vi "PopulateControlsFromCSV-OLD.vi"() -> ()   [LabVIEW 2019]
uses:
  <vilib>/Utility/file.llb/Read Delimited Spreadsheet (string).vi
panel:
  out "Boolean":bool
  out "number":dbl
  out "element":string
  out "index of element":i32
  out "Label.Text":string="all rows"
  out "all rows":string[][](array[string])
  in  "Numeric4":dbl
  in  "Numeric3":dbl
  in  "Numeric2":dbl
  in  "Numeric1":dbl
  in  "Path":path=path "C:/Users/jbrus/Documents/GitHub/LabVIEW/3LabVIEWFeatures/PopulateControlsFromCSV/FileOutput.csv"
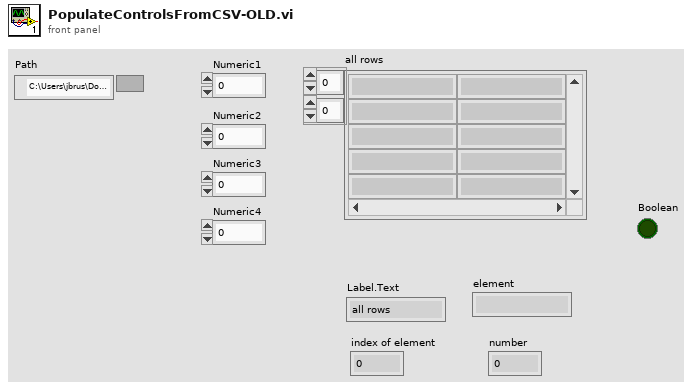
[diagram p1: front panel]
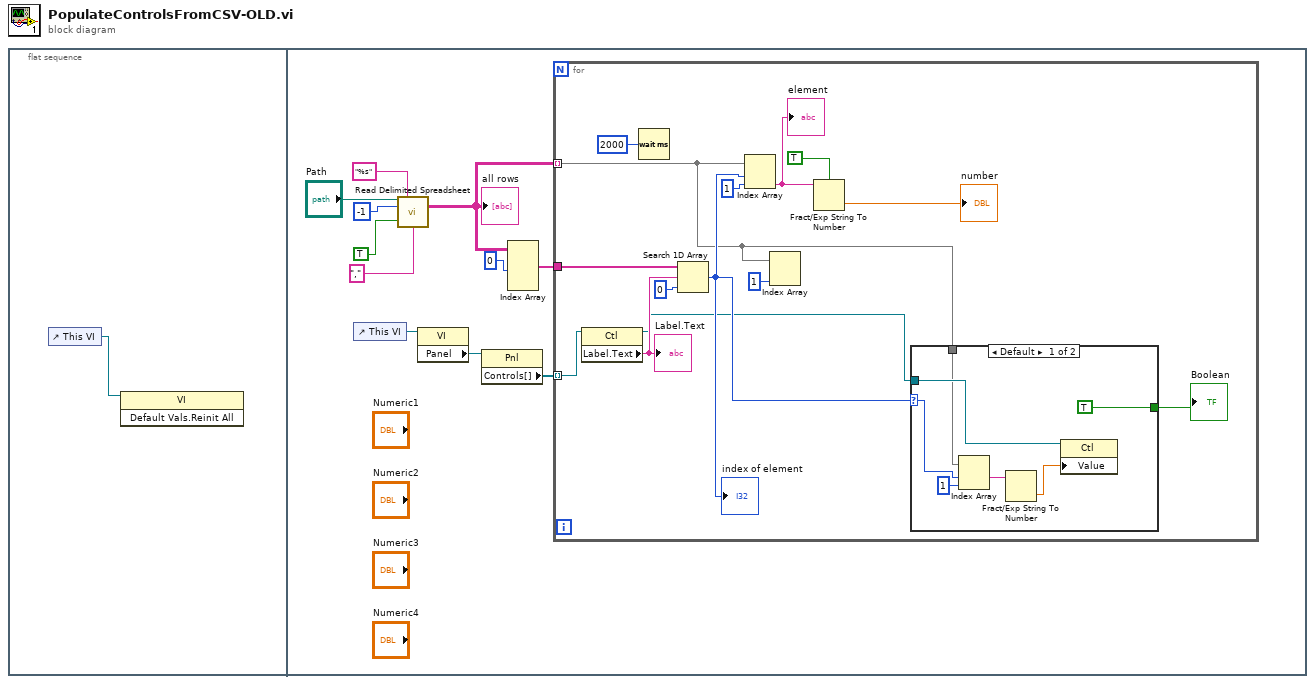
[diagram p0: block diagram]
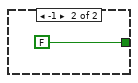
[diagram p2: hidden frame]
diagram:
  n1 = flat-sequence {
    frame #0 {
      n2 = control-ref of="This VI"() -> (w1:refnum<vi>)
      n3 = invoke class="VI" method="Default Vals.Reinit All"(reference=w1) -> ()  [unwired: 2 in, 3 out]
    }
    frame #1 {
      n4 = control-ref of="This VI"() -> (w7:refnum<vi>)
      n5 = call-poly <vilib>:"Read Delimited Spreadsheet.vi"("file path (dialog if empty)"="Path", "format (%s)"="%s", "number of rows (all:-1)"=-1, "transpose? (F)"=TRUE, "delimiter (\\t)"="," ("delimiter (\\t)")) -> ("all rows"=w12:string[][])  [unwired: 5 in, 5 out]
      "all rows" <- w12
      n6 = property class="VI"(reference=w7) -> ("Panel"=w8:refnum<vi>)  [unwired: 1 in, 2 out]
      n7 = property class="Pnl"(reference=w8) -> ("Controls[]"=w9:refnum<vi>[])  [unwired: 1 in, 2 out]
      n8 = Index Array(array=w12, index (col) #1=0 ("index")) -> (element #1=w11:string[])  [unwired: 3 in, 1 out]
      n9 = for {
        tunnel: w9 -> [w16] mode=indexing
        tunnel: w11 -> [w24]
        tunnel: w12 -> [w14] mode=indexing
        n10 = property class="Ctl"(reference=w16) -> (reference out=w13:refnum<vi>, "Label.Text"=w23:string)  [unwired: 1 in, 1 out]
        "Label.Text" <- w23
        n11 = Wait (ms)(milliseconds to wait=u32 2000) -> ()  [unwired: 1 out]
        n12 = Search 1D Array(1D array=w24, element=w23, start index (0)=0) -> (index of element=w18:i32)
        "index of element" <- w18
        n13 = Index Array(array=w14, index #1=w18, index #2=1 ("index")) -> (element #2=w20:string)  [unwired: 1 out]
        "element" <- w20
        n14 = Index Array(array=w14, index #2=1 ("index")) -> ()  [unwired: 1 in, 2 out]
        n15 = Fract/Exp String To Number(use system decimal point (T)=TRUE, string=w20) -> (number=→"number":dbl)  [unwired: 2 in, 1 out]
        n16 = case shown="Default" w18 {
          selector: w18 -> [w29 _]
          tunnel: [TRUE FALSE] -> w17
          tunnel: w13 -> [w32 _]
          tunnel: w14 -> [w31 _]
          frame Default {
            n17 = Index Array(array=w31, index #1=w29, index #2=1 ("index")) -> (element #1=w28:string)  [unwired: 1 out]
            n18 = Fract/Exp String To Number(string=w28) -> (number=w27:dbl)  [unwired: 3 in, 1 out]
            n19 = property class="Ctl"(reference=w32, "Value"=w27) -> ()  [unwired: 1 in, 2 out]
          }
          frame -1 {
          }
        }
        "Boolean" <- w17
      }
    }
  }
